vi "Parse Color.vi"(10 "error in (no error)":errorcluster, 11 "Color String":string) -> (2 "error out":errorcluster, 3 "Color":u32(colorbox))   [LabVIEW 2020, in "VolatusGUIElements.lvlib" / "DblStatusIndicator.lvclass"]
uses:
  DblStatusIndicator.lvclass
  DblStatusIndicator.lvclass/DblStatusIndicator.ctl
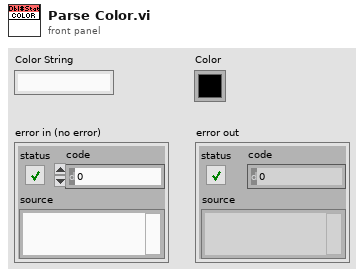
[diagram p1: front panel]
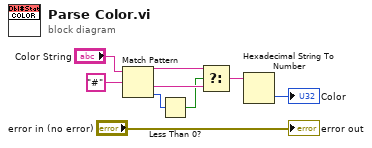
[diagram p0: block diagram]
diagram:
  n1 = Match Pattern(string="Color String", regular expression="#") -> (before substring=w6:string, after substring=w5:string, offset past match=w7:i32)  [unwired: 1 in, 1 out]
  n2 = Less Than 0?(x=w7) -> (x < 0?=w4:bool)
  n3 = Select(t=w6, s=w4, f=w5) -> (s? t:f=w3:string)
  n4 = Hexadecimal String To Number(string=w3) -> (number=→"Color":u32)  [unwired: 2 in, 1 out]
  "error out" <- "error in (no error)"
